vi "Non Linear PID Controller.vi"   [LabVIEW 2014, in "Controller Library.lvlib" / "Non Linear PID Controller.lvclass"]
uses:
  Non Linear PID Controller.lvclass
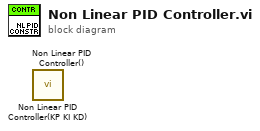
[diagram p0: block diagram]
diagram:
  n1 = call "Non Linear PID Controller(KP KI KD).vi"() -> ()  [unwired: 11 in, 1 out]
  n2 = call "Non Linear PID Controller().vi"() -> ()  [unwired: 11 in, 1 out]
